vi "Exclude Polymorphic VIs.vi"(7 "Exclude ?":bool, 8 "error in (no error)":errorcluster, 11 "BuildSpec in":refnum<vi>) -> (0 "error out":errorcluster, 3 "BuildSpec out":refnum<vi>)   [LabVIEW 2019, in "Project Sync Tools.lvclass"]
uses:
  Project Sync Tools.lvclass
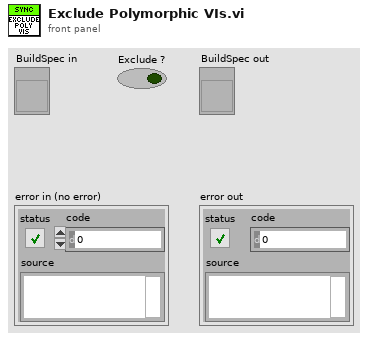
[diagram p1: front panel]
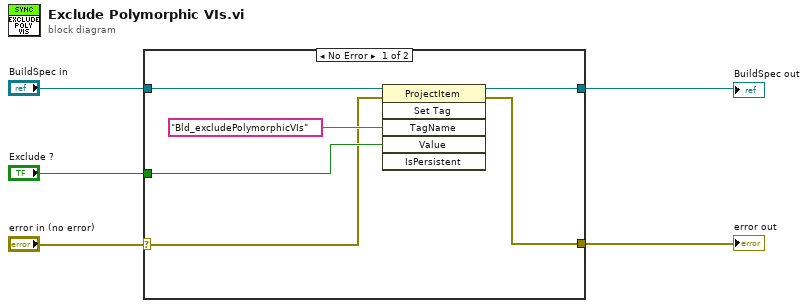
[diagram p0: block diagram]
diagram:
  n1 = case shown="No Error" "error in (no error)" {
    selector: "error in (no error)" -> [w6 w12]
    tunnel: [w11 w12] -> w5
    tunnel: [w10 w13] -> w4
    tunnel: "BuildSpec in" -> [w9 w13]
    tunnel: "Exclude ?" -> [w8 _]
    frame No Error {
      n2 = invoke class="ProjectItem" method="Set Tag"(reference=w9, error in=w6, "TagName"="Bld_excludePolymorphicVIs" ("Tag Name"), "Value"=w8) -> (reference out=w10:refnum<vi>, error out=w11:errorcluster)  [unwired: 2 in, 4 out]
    }
    frame Error {
    }
  }
  "error out" <- w5
  "BuildSpec out" <- w4
